vi "openbci_reset_register.vi"(8 "error in (no error)":errorcluster, 11 "OBCI dev in":T1={"COM port"="", "n_ch (8)"=enum."8 Channels", "delay_tx"=50}) -> (0 "error out":errorcluster, 2 "reset_reg_str":string, 3 "OBCI dev out":T1={"COM port"="", "n_ch (8)"=enum."8 Channels", "delay_tx"=50})   [LabVIEW 2013]
doc: "Reseting OpenBCI registers to default"
uses:
  Control Def/openbci_device.ctl
  Control Def/channel_count.ctl
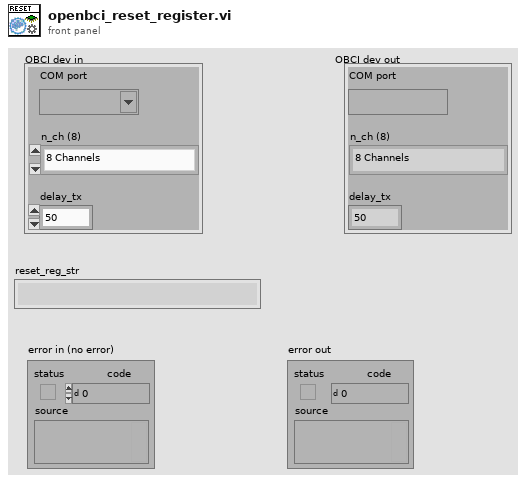
[diagram p1: front panel]
types:
  T1 = typedef "openbci_device.ctl" = cluster{"COM port":refnum<visa-resource-name>, "n_ch (8)":T2, "delay_tx":u32}
  T2 = typedef "channel_count.ctl" = enum16{"8 Channels", "16 Channels"}
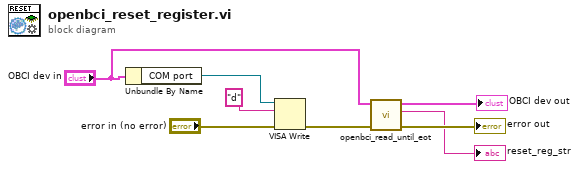
[diagram p0: block diagram]
diagram:
  n1 = Unbundle By Name("OBCI dev in") -> ("COM port"=w3:refnum<visa-resource-name>)
  n2 = VISA Write(VISA resource name=w3, write buffer="d", error in (no error)="error in (no error)") -> (error out=w6:errorcluster)  [unwired: 2 out]
  n3 = call "openbci_read_until_eot.vi"("error in"=w6, "OBCI dev in"="OBCI dev in") -> ("error out"=→"error out":errorcluster, "string"=→"reset_reg_str":string, "OBCI dev out"=→"OBCI dev out":T1)  [unwired: 7 in]
